vi "Actor Core.vi"(8 "error in":errorcluster, 11 "Child_5_Class in":refnum<class "Error_Emgime_Class.lvclass">) -> (0 "error out":errorcluster, 3 "Actor out":refnum<class "Actor.lvclass">)   [LabVIEW 2023, in "Error_Engine_Actor.lvlib" / "Error_Emgime_Class.lvclass"]
doc: "(<B>Filename</B>: Actor Framework.lvlib:Actor.lvclass:Actor Core.vi)\n\nReceives messages to the actor, reacts to them, and initiates any error handling that may shut the actor down.\n\nDescendant classes may override this VI to append parallel tasks for the actor to complete while it handles messages. Overrides use the Call Parent Class Method node."
uses:
  Error_Emgime_Class.lvclass
  <vilib>/ActorFramework/Actor/Actor.lvclass
  Abstraction_Interface_Class/Abstraction_Interface_Class.lvclass
panel:
  out "RAW_Actor_Name":string
  in  "Console":string
  # "Error Engine"
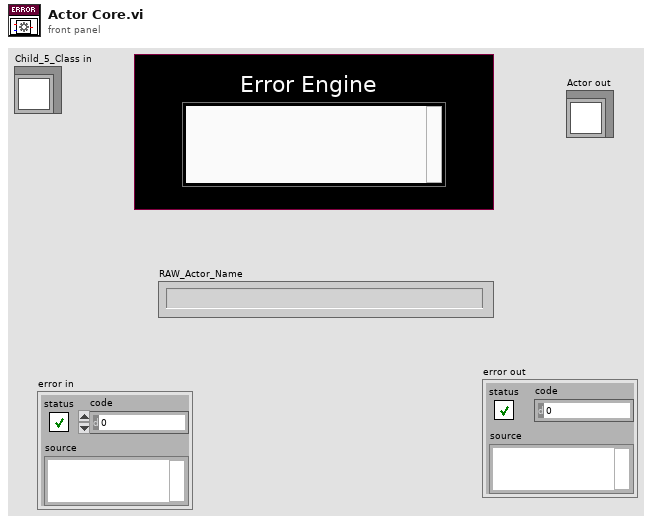
[diagram p1: front panel]
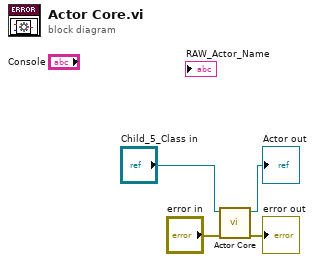
[diagram p0: block diagram]
diagram:
  n1 = call-parent "Actor Core.vi"("error in"="error in", "Actor in"="Child_5_Class in") -> ("error out"=→"error out":errorcluster, "Actor out"=→"Actor out":refnum<class "Actor.lvclass">)  [unwired: 8 in]
